vi "FrontPannelExample.vi"(0 "End Session":bool) -> (1 "Properties from ThingWorx":string[][](array[string])=[["Button", "true"], ["Button2", "true"], ["description", ""], ["isConnected", "false"], ["lastConnection", "1970-01-01T00:00:00.000Z"], ["name", "GenericEdge"], ["Photocell", "200.0"], ["Potentiometer", "234.0"], ["tags", "GenericRemoteEdge:Example"], ["Temperature", "0.242"], ["thingTemplate", "GenericThingTemplate"]])   [LabVIEW 2015]
uses:
  <vilib>/httpClient/LabVIEWHTTPClient.lvlib
panel:
  in  "Thermometer":dbl(slide) scale=0.0..100.0
  in  "Potentiometer":dbl(knob) scale=0.0..500.0
  in  "Photocell Intensity":dbl(slide) scale=0.0..500.0
  in  "Button2":bool
  in  "Button":bool
  out "error out":errorcluster
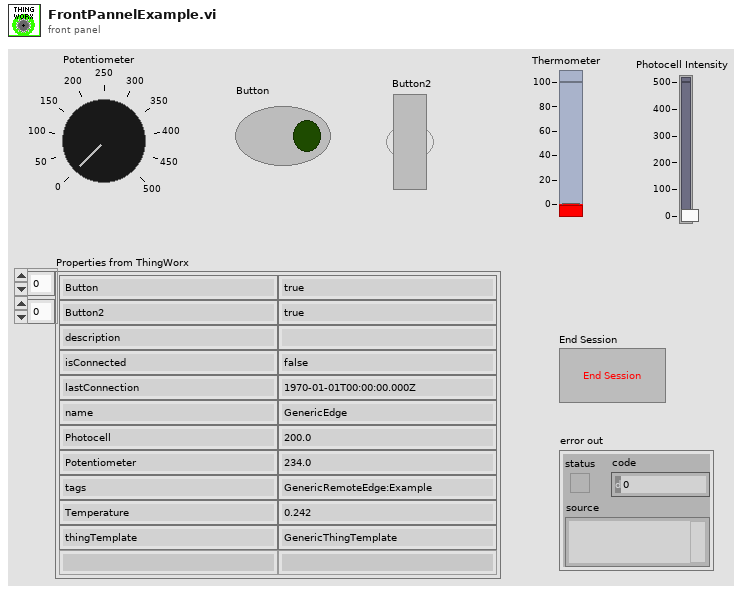
[diagram p1: front panel]
types:
  T1 = typedef "LabVIEWHTTPClient.lvlib/ClientHandle.ctl" = refnum<k1>
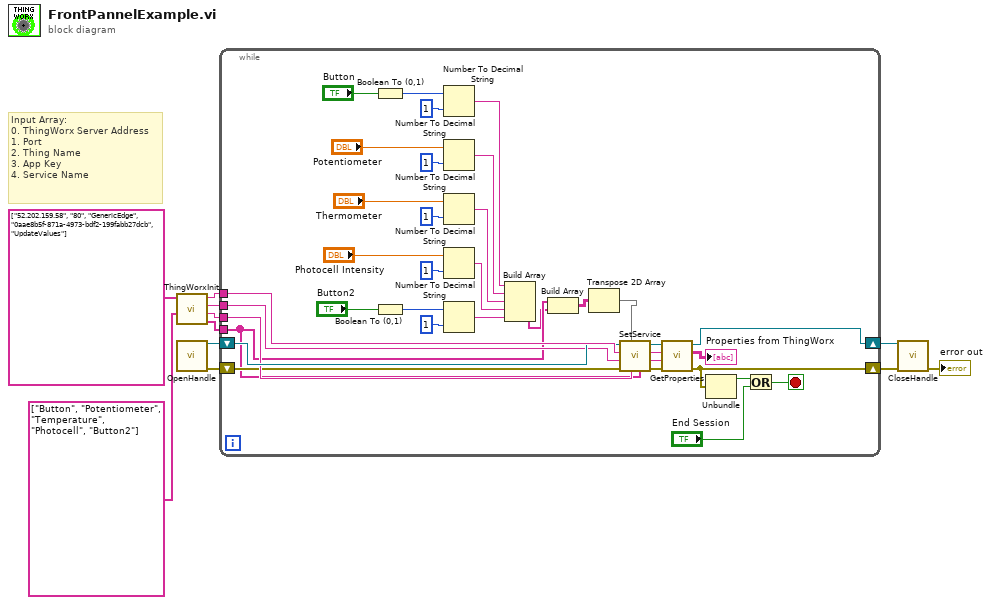
[diagram p0: block diagram]
diagram:
  # "Input Array:\n0. ThingWorx Server Address\n1. Port\n2. Thing Name\n3. App Key\n4. Service Name"
  n1 = call "ThingWorxInit.vi"("Properties"=string[] ["Button", "Potentiometer", "Temperature", "Photocell", "Button2"] ("Properties in Service"), "Input Array"=string[] ["52.202.159.58", "80", "GenericEdge", "0aae8b5f-871a-4973-bdf2-199fabb27dcb", "UpdateValues"]) -> ("Properties Out"=w1:string[], "Service Name"=w3:string, "appKey"=w10:string, "url beginning"=w11:string)  [unwired: 6 in]
  n2 = call <vilib>:"OpenHandle.vi"() -> ("client handle out"=w6:T1, "error out"=w5:errorcluster)  [unwired: 14 in]
  n3 = while {
    tunnel: w11 -> [w43]
    shift-right: [w47] -> w8
    shift-left: w6 -> [w42]
    shift-right: [w34] -> w9
    shift-left: w5 -> [w33]
    tunnel: w10 -> [w41]
    tunnel: w3 -> [w36]
    tunnel: w1 -> [w13]
    stop <- w46 stop-if-true
    n4 = Boolean To (0,1)(Boolean="Button") -> (0, 1=w27:i16)
    n5 = Boolean To (0,1)(Boolean="Button2") -> (0, 1=w29:i16)
    n6 = Number To Decimal String(number=w27, width (-)=i16 1) -> (decimal integer string=w26:string)
    n7 = Number To Decimal String(number="Potentiometer", width (-)=i16 1) -> (decimal integer string=w19:string)
    n8 = Number To Decimal String(number="Thermometer", width (-)=i16 1) -> (decimal integer string=w16:string)
    n9 = Number To Decimal String(number="Photocell Intensity", width (-)=i16 1) -> (decimal integer string=w22:string)
    n10 = Number To Decimal String(number=w29, width (-)=i16 1) -> (decimal integer string=w25:string)
    n11 = Build Array(w26, w19, w16, w22, w25) -> (w12:string[])
    n12 = Build Array(w13, w12) -> (w15:string[][])
    n13 = Transpose 2D Array(2D array=w15) -> (transposed array=w14:string[][])
    n14 = call "SetService.vi"("Properties in Service"=w13, "Service Name"=w36, "Properties"=w14, "error in"=w33, "appKey"=w41, "uri beginning"=w43, "client handle"=w42) -> ("error out"=w35:errorcluster, "appKey out"=w38:string, "uri beginning out"=w37:string, "client handle out"=w39:T1)  [unwired: 1 out]
    n15 = call "GetProperties.vi"("error in (no error)"=w35, "appKey"=w38, "url beginning"=w37, "client handle"=w39) -> ("error out"=w34:errorcluster, "Array"=→"Properties from ThingWorx":string[][], "client handle out"=w47:T1)  [unwired: 3 in, 2 out]
    n16 = Unbundle(w34) -> ("status"=w44:bool)  [unwired: 2 out]
    n17 = Or(x=w44, y="End Session") -> (x .or. y?=w46:bool)
  }
  n18 = call <vilib>:"CloseHandle.vi"("client handle"=w8, "error in (no error)"=w9) -> ("error out"=→"error out":errorcluster)  [unwired: 13 in]
